vi "gyro-pll-V3.vi"() -> ()   [LabVIEW 2018]
uses:
  lorentzian.ctl
  circle corners.ctl
  pid -- parameters.ctl
  <vilib>/event_ctls.llb/eventvkey.ctl
  show-win- control.ctl
  PID - mode.ctl
  pll parameters.ctl
  server talk-to-back pair.ctl
  server talkback message type.ctl
  server talkto message type.ctl
  agregator -- action.ctl
  interpolation state - real.ctl
  pll internal user event action.ctl
  publisher action.ctl
  four-corner circle transformation.ctl
  cursor action.ctl
  Q -- check range -- i -- real.vi
  linear interpolation - real.vi
  draw a circle.vi
  linear interpolation iiii- complex.vi
  <vilib>/Analysis/baseanly.llb/A x B.vi
  <vilib>/Analysis/baseanly.llb/Complex A x B.vi
  line -- complex.vi
  Q -- check range -- i -- integer.vi
  generate linear region.vi
  Q - not nan -- real.vi
  Q - not nan -- integer.vi
  <vilib>/Analysis/Matrix/Numeric/Conversions/Array To Matrix.vi
  <vilib>/Analysis/Matrix/Numeric/Conversions/Array To Matrix - RA2.vi
  <vilib>/Analysis/baseanly.llb/Inverse Matrix.vi
  <vilib>/Analysis/baseanly.llb/Real Inverse Matrix.vi
panel:
  in  "(*) sweeper server":bool=TRUE
  in  "(*) pll":bool
  in  "exit!":bool
  in  "(*) sourcer":bool
  in  "(*) fitter":bool
  in  "(*) sweeper":bool=TRUE
  in  "PID parameters :{}[];'":T1={"I (sec)"=0.004634123928756344, "P (sec)"=0.008980860327047186} {"P (sec)" scale=0.01..10.0; "I (sec)" scale=0.01..10.0}
  in  "PLL ON":bool
  in  "stop pll async":bool
  in  "start pll async":bool
  in  "pll parameters":T2={"PID parameters"={"I (sec)"=0.004634123928756344, "P (sec)"=0.008980860327047186}, "PID mode"=enum."normal", "plot hist time (sec)"=1.0, "dt (sec)"=0.001, "visc hist time (sec)"=2.0, "time int ave time (sec)"=0.3, "PLL limits (Hz)"=5000.0} {"PLL limits (Hz)" format="%#.2f"; "time int ave time (sec)" format="%#_10f"; "visc hist time (sec)" format="%#_10f"; "dt (sec)" format="%#_10f"; "plot hist time (sec)" format="%#_10f"; "PID parameters"."P (sec)" scale=0.01..10.0; "PID parameters"."I (sec)" scale=0.01..10.0}
  in  "all 3":T4(tab)
  in  "reset lorentzian! :q":bool
  in  "Tab Control":enum32{"PID", "hist", "params"}(tab)=enum."params"
  out "Plot: complex- hist":cluster{dbl[], dbl[]}[](graph)=[{array[1000 elements], array[1000 elements]}, {[7.190597353205284e-06, 7.172141018125027e-06, 7.116804391567491e-06, 7.024684552779172e-06, 6.895943111259833e-06, 6.7308059232445354e-06, 6.529562695475053e-06, 6.292566476955803e-06, 6.020233039585921e-06, 5.713040148754082e-06, 5.371526725175644e-06, 4.996291899442611e-06, 4.5879939609449636e-06, 4.147349203007406e-06, 3.6751306662674513e-06, 3.1721667824994774e-06, 2.6393399212638878e-06, 2.0775848419310813e-06, 1.4878870537958579e-06, 8.712810871592677e-07, 2.2884867841089993e-07, -4.382831277042918e-07, -1.1289439553054788e-06, -1.8419221506129192e-06, -2.575966907600425e-06, -3.329790462334158e-06, -4.102070352148148e-06, -4.891451735693187e-06, -5.696549769788949e-06, -6.515952038909475e-06, -7.348221033039968e-06, -8.191896669557811e-06, -9.045498854713654e-06, -9.907530080218758e-06, -1.0776478050383408e-05, -1.1650818335197432e-05, -1.252901704469844e-05, -1.3409533519936043e-05, -1.4290823035811157e-05, -1.5171339511048758e-05, -1.6049538220549768e-05, -1.692387850536379e-05, -1.7792826475528438e-05, -1.8654857701033543e-05, -1.950845988618939e-05, -2.035213552270723e-05, -2.1184404516837726e-05, -2.200380678595825e-05, -2.2808904820054008e-05, -2.3598286203599055e-05, -2.4370566093413044e-05, -2.5124389648146775e-05, -2.5858434405134282e-05, -2.6571412600441725e-05, -2.7262073428042906e-05, -2.79292052341581e-05, -2.8571637642906468e-05, -2.918824360954306e-05, -2.9777941397678286e-05, -3.0339696477011096e-05, -3.087252333824668e-05, -3.137548722201465e-05, -3.184770575875461e-05, -3.228835051669217e-05, -3.269664845518981e-05, -3.3071883280922845e-05, -3.341339670450129e-05, -3.372058959533313e-05, -3.399292303270301e-05, -3.4229919251222255e-05, -3.4431162478991744e-05, -3.4596299667007035e-05, -3.472504110852638e-05, -3.4817160947314696e-05, -3.4872497573872235e-05, -3.489095390895249e-05, -3.4872497573872235e-05, -3.4817160947314696e-05, -3.472504110852638e-05, -3.459629966700704e-05, -3.4431162478991744e-05, -3.422991925122226e-05, -3.3992923032703014e-05, -3.372058959533313e-05, -3.341339670450129e-05, -3.307188328092285e-05, -3.269664845518982e-05, -3.2288350516692175e-05, -3.1847705758754615e-05, -3.137548722201466e-05, -3.087252333824669e-05, -3.0339696477011103e-05, -2.9777941397678293e-05, -2.9188243609543066e-05, -2.8571637642906474e-05, -2.7929205234158112e-05, -2.726207342804292e-05, -2.6571412600441735e-05, -2.5858434405134296e-05, -2.512438964814679e-05, -2.4370566093413057e-05, -2.3598286203599066e-05, -2.280890482005402e-05, -2.200380678595826e-05, -2.1184404516837737e-05, -2.035213552270724e-05, -1.9508459886189396e-05, -1.865485770103357e-05, -1.7792826475528462e-05, -1.6923878505363813e-05, -1.6049538220549788e-05, -1.5171339511048779e-05, -1.4290823035811176e-05, -1.3409533519936056e-05, -1.2529017044698455e-05, -1.1650818335197446e-05, -1.0776478050383421e-05, -9.907530080218769e-06, -9.045498854713664e-06, -8.19189666955782e-06, -7.348221033039972e-06, -6.515952038909498e-06, -5.69654976978897e-06, -4.891451735693207e-06, -4.102070352148165e-06, -3.3297904623341733e-06, -2.575966907600442e-06, -1.8419221506129327e-06, -1.1289439553054907e-06, -4.3828312770430365e-07, 2.2884867841089146e-07, 8.712810871592576e-07, 1.4878870537958511e-06, 2.0775848419310745e-06, 2.6393399212638844e-06, 3.172166782499474e-06, 3.6751306662674378e-06, 4.147349203007396e-06, 4.587993960944957e-06, 4.996291899442601e-06, 5.371526725175637e-06, 5.713040148754075e-06, 6.020233039585914e-06, 6.292566476955799e-06, 6.52956269547505e-06, 6.7308059232445354e-06, 6.89594311125983e-06, 7.024684552779168e-06, 7.116804391567491e-06, 7.172141018125027e-06], [0.0002113633008955132, 0.00021224439713003404, 0.00021312394762236102, 0.00021400040934205735, 0.00021487224467744295, 0.00021573792413308792, 0.00021659592901306725, 0.0002174447540852694, 0.00021828291022208502, 0.0002191089270128428, 0.00021992135534340933, 0.00022071876993842783, 0.00022149977186173528, 0.00022226299097057205, 0.00022300708831927754, 0.00022373075850825623, 0.00022443273197409182, 0.00022511177721679307, 0.00022576670296026313, 0.00022639636024220273, 0.00022699964442978034, 0.0002275754971575336, 0.000228122908184102, 0.00022864091716453335, 0.0002291286153350554, 0.0002295851471073561, 0.00023000971156957625, 0.00023040156389138116, 0.0002307600166306461, 0.00023108444093946333, 0.00023137426766735506, 0.00023162898835975677, 0.0002318481561500193, 0.00023203138654336486, 0.0002321783580914214, 0.00023228881295615236, 0.00023236255736219216, 0.00023239946193679412, 0.00023239946193679412, 0.00023236255736219216, 0.00023228881295615236, 0.0002321783580914214, 0.00023203138654336486, 0.0002318481561500193, 0.00023162898835975677, 0.00023137426766735506, 0.00023108444093946333, 0.00023076001663064613, 0.00023040156389138116, 0.00023000971156957625, 0.0002295851471073561, 0.0002291286153350554, 0.00022864091716453335, 0.000228122908184102, 0.0002275754971575336, 0.00022699964442978034, 0.00022639636024220273, 0.00022576670296026315, 0.00022511177721679307, 0.00022443273197409182, 0.00022373075850825623, 0.00022300708831927757, 0.00022226299097057205, 0.0002214997718617353, 0.00022071876993842783, 0.00021992135534340933, 0.0002191089270128428, 0.00021828291022208502, 0.0002174447540852694, 0.00021659592901306725, 0.00021573792413308792, 0.00021487224467744295, 0.00021400040934205735, 0.00021312394762236102, 0.00021224439713003404, 0.0002113633008955132, 0.00021048220466099237, 0.0002096026541686654, 0.0002087261924489691, 0.0002078543571135835, 0.0002069886776579385, 0.00020613067277795916, 0.00020528184770575705, 0.00020444369156894142, 0.00020361767477818362, 0.00020280524644761708, 0.0002020078318525986, 0.00020122682992929113, 0.0002004636108204544, 0.00019971951347174887, 0.00019899584328277018, 0.0001982938698169346, 0.00019761482457423337, 0.0001969598988307633, 0.00019633024154882368, 0.00019572695736124607, 0.0001951511046334928, 0.00019460369360692445, 0.00019408568462649307, 0.00019359798645597102, 0.00019314145468367035, 0.0001927168902214502, 0.00019232503789964525, 0.0001919665851603803, 0.00019164216085156309, 0.00019135233412367135, 0.00019109761343126964, 0.0001908784456410071, 0.00019069521524766155, 0.000190548243699605, 0.00019043778883487406, 0.00019036404442883425, 0.0001903271398542323, 0.0001903271398542323, 0.00019036404442883425, 0.00019043778883487406, 0.000190548243699605, 0.00019069521524766155, 0.0001908784456410071, 0.00019109761343126964, 0.00019135233412367135, 0.00019164216085156306, 0.00019196658516038029, 0.00019232503789964523, 0.00019271689022145016, 0.00019314145468367033, 0.000193597986455971, 0.00019408568462649307, 0.00019460369360692443, 0.0001951511046334928, 0.00019572695736124607, 0.00019633024154882368, 0.00019695989883076326, 0.00019761482457423334, 0.0001982938698169346, 0.00019899584328277018, 0.00019971951347174885, 0.00020046361082045436, 0.0002012268299292911, 0.00020200783185259858, 0.00020280524644761705, 0.0002036176747781836, 0.0002044436915689414, 0.00020528184770575702, 0.00020613067277795916, 0.0002069886776579385, 0.00020785435711358346, 0.00020872619244896907, 0.00020960265416866537, 0.00021048220466099237]}, {[7.168586400274939e-06, 5.066709932460086e-06, 2.964833464645231e-06, 8.629569968303764e-07, -1.2389194709844774e-06, -3.340795938799331e-06, -5.442672406614187e-06, -7.54454887442904e-06, -9.646425342243894e-06, -1.174830181005875e-05, -1.3850178277873602e-05, -1.5952054745688457e-05, -1.8053931213503313e-05, -2.0155807681318165e-05, -2.225768414913302e-05, -2.4359560616947872e-05, -2.6461437084762728e-05, -2.8563313552577583e-05, -3.066519002039244e-05, -3.276706648820729e-05], [0.00021232547061132137, 0.00021222925363974056, 0.00021213303666815973, 0.00021203681969657892, 0.0002119406027249981, 0.0002118443857534173, 0.00021174816878183648, 0.00021165195181025565, 0.00021155573483867484, 0.000211459517867094, 0.0002113633008955132, 0.0002112670839239324, 0.00021117086695235157, 0.00021107464998077076, 0.00021097843300918993, 0.00021088221603760913, 0.00021078599906602832, 0.0002106897820944475, 0.00021059356512286668, 0.00021049734815128585]}, {[-1.288800856206544e-05, -1.2984225533646258e-05, -1.3080442505227073e-05, -1.317665947680789e-05, -1.3272876448388706e-05, -1.3369093419969523e-05, -1.3465310391550338e-05, -1.3561527363131155e-05, -1.365774433471197e-05, -1.3753961306292788e-05, -1.3850178277873605e-05, -1.394639524945442e-05, -1.4042612221035236e-05, -1.4138829192616053e-05, -1.423504616419687e-05, -1.4331263135777686e-05, -1.4427480107358503e-05, -1.4523697078939318e-05, -1.4619914050520135e-05, -1.471613102210095e-05], [0.00019034453621736468, 0.00019244641268517952, 0.0001945482891529944, 0.00019665016562080923, 0.0001987520420886241, 0.00020085391855643894, 0.00020295579502425378, 0.00020505767149206865, 0.0002071595479598835, 0.00020926142442769836, 0.0002113633008955132, 0.00021346517736332805, 0.00021556705383114292, 0.00021766893029895776, 0.00021977080676677263, 0.00022187268323458747, 0.0002239745597024023, 0.00022607643617021718, 0.00022817831263803202, 0.0002302801891058469]}, {[9.092925831891258e-06, 8.900491888729626e-06, 8.708057945567993e-06, 8.515624002406362e-06, 8.32319005924473e-06, 8.130756116083097e-06, 7.938322172921465e-06, 7.745888229759832e-06, 7.5534542865982e-06, 7.361020343436568e-06, 7.168586400274936e-06, 6.976152457113303e-06, 6.783718513951671e-06, 6.591284570790038e-06, 6.3988506276284065e-06, 6.206416684466774e-06, 6.013982741305142e-06, 5.82154879814351e-06, 5.629114854981877e-06, 5.4366809118202445e-06], [0.0001702879412550243, 0.00017449169419065402, 0.00017869544712628373, 0.00018289920006191342, 0.00018710295299754313, 0.00019130670593317284, 0.00019551045886880255, 0.00019971421180443226, 0.00020391796474006197, 0.00020812171767569168, 0.00021232547061132137, 0.00021652922354695108, 0.0002207329764825808, 0.0002249367294182105, 0.0002291404823538402, 0.0002333442352894699, 0.00023754798822509963, 0.00024175174116072932, 0.00024595549409635905, 0.00025015924703198874]}, {[-1.97103396318906e-05, -1.91243234964889e-05, -1.8538307361087202e-05, -1.79522912256855e-05, -1.73662750902838e-05, -1.6780258954882103e-05, -1.6194242819480402e-05, -1.5608226684078704e-05, -1.5022210548677003e-05, -1.4436194413275303e-05, -1.3850178277873603e-05, -1.3264162142471904e-05, -1.2678146007070203e-05, -1.2092129871668504e-05, -1.1506113736266805e-05, -1.0920097600865104e-05, -1.0334081465463405e-05, -9.748065330061706e-06, -9.162049194660005e-06, -8.576033059258306e-06], [0.00023375398508080204, 0.00023151491666227315, 0.00022927584824374426, 0.0002270367798252154, 0.0002247977114066865, 0.00022255864298815762, 0.00022031957456962873, 0.00021808050615109985, 0.00021584143773257098, 0.0002136023693140421, 0.0002113633008955132, 0.00020912423247698432, 0.00020688516405845543, 0.00020464609563992657, 0.00020240702722139768, 0.0002001679588028688, 0.0001979288903843399, 0.00019568982196581104, 0.00019345075354728215, 0.00019121168512875326]}]
  in  "dt (sec)":dbl=0.001 format="%#_10f"
  in  "plot hist time (sec)":dbl=1.0 format="%#_10f"
  in  "PID mode":T3
  out "G (Hz)":dbl=6.817921124952451 format="%#.4f"
  in  "reset freq! :r":bool
  out "Plot: complex plane":cluster{dbl[], dbl[]}[](graph)=[{[7.190597353205284e-06, 7.172141018125027e-06, 7.116804391567491e-06, 7.024684552779172e-06, 6.895943111259833e-06, 6.7308059232445354e-06, 6.529562695475053e-06, 6.292566476955803e-06, 6.020233039585921e-06, 5.713040148754082e-06, 5.371526725175644e-06, 4.996291899442611e-06, 4.5879939609449636e-06, 4.147349203007406e-06, 3.6751306662674513e-06, 3.1721667824994774e-06, 2.6393399212638878e-06, 2.0775848419310813e-06, 1.4878870537958579e-06, 8.712810871592677e-07, 2.2884867841089993e-07, -4.382831277042918e-07, -1.1289439553054788e-06, -1.8419221506129192e-06, -2.575966907600425e-06, -3.329790462334158e-06, -4.102070352148148e-06, -4.891451735693187e-06, -5.696549769788949e-06, -6.515952038909475e-06, -7.348221033039968e-06, -8.191896669557811e-06, -9.045498854713654e-06, -9.907530080218758e-06, -1.0776478050383408e-05, -1.1650818335197432e-05, -1.252901704469844e-05, -1.3409533519936043e-05, -1.4290823035811157e-05, -1.5171339511048758e-05, -1.6049538220549768e-05, -1.692387850536379e-05, -1.7792826475528438e-05, -1.8654857701033543e-05, -1.950845988618939e-05, -2.035213552270723e-05, -2.1184404516837726e-05, -2.200380678595825e-05, -2.2808904820054008e-05, -2.3598286203599055e-05, -2.4370566093413044e-05, -2.5124389648146775e-05, -2.5858434405134282e-05, -2.6571412600441725e-05, -2.7262073428042906e-05, -2.79292052341581e-05, -2.8571637642906468e-05, -2.918824360954306e-05, -2.9777941397678286e-05, -3.0339696477011096e-05, -3.087252333824668e-05, -3.137548722201465e-05, -3.184770575875461e-05, -3.228835051669217e-05, -3.269664845518981e-05, -3.3071883280922845e-05, -3.341339670450129e-05, -3.372058959533313e-05, -3.399292303270301e-05, -3.4229919251222255e-05, -3.4431162478991744e-05, -3.4596299667007035e-05, -3.472504110852638e-05, -3.4817160947314696e-05, -3.4872497573872235e-05, -3.489095390895249e-05, -3.4872497573872235e-05, -3.4817160947314696e-05, -3.472504110852638e-05, -3.459629966700704e-05, -3.4431162478991744e-05, -3.422991925122226e-05, -3.3992923032703014e-05, -3.372058959533313e-05, -3.341339670450129e-05, -3.307188328092285e-05, -3.269664845518982e-05, -3.2288350516692175e-05, -3.1847705758754615e-05, -3.137548722201466e-05, -3.087252333824669e-05, -3.0339696477011103e-05, -2.9777941397678293e-05, -2.9188243609543066e-05, -2.8571637642906474e-05, -2.7929205234158112e-05, -2.726207342804292e-05, -2.6571412600441735e-05, -2.5858434405134296e-05, -2.512438964814679e-05, -2.4370566093413057e-05, -2.3598286203599066e-05, -2.280890482005402e-05, -2.200380678595826e-05, -2.1184404516837737e-05, -2.035213552270724e-05, -1.9508459886189396e-05, -1.865485770103357e-05, -1.7792826475528462e-05, -1.6923878505363813e-05, -1.6049538220549788e-05, -1.5171339511048779e-05, -1.4290823035811176e-05, -1.3409533519936056e-05, -1.2529017044698455e-05, -1.1650818335197446e-05, -1.0776478050383421e-05, -9.907530080218769e-06, -9.045498854713664e-06, -8.19189666955782e-06, -7.348221033039972e-06, -6.515952038909498e-06, -5.69654976978897e-06, -4.891451735693207e-06, -4.102070352148165e-06, -3.3297904623341733e-06, -2.575966907600442e-06, -1.8419221506129327e-06, -1.1289439553054907e-06, -4.3828312770430365e-07, 2.2884867841089146e-07, 8.712810871592576e-07, 1.4878870537958511e-06, 2.0775848419310745e-06, 2.6393399212638844e-06, 3.172166782499474e-06, 3.6751306662674378e-06, 4.147349203007396e-06, 4.587993960944957e-06, 4.996291899442601e-06, 5.371526725175637e-06, 5.713040148754075e-06, 6.020233039585914e-06, 6.292566476955799e-06, 6.52956269547505e-06, 6.7308059232445354e-06, 6.89594311125983e-06, 7.024684552779168e-06, 7.116804391567491e-06, 7.172141018125027e-06], [0.0002113633008955132, 0.00021224439713003404, 0.00021312394762236102, 0.00021400040934205735, 0.00021487224467744295, 0.00021573792413308792, 0.00021659592901306725, 0.0002174447540852694, 0.00021828291022208502, 0.0002191089270128428, 0.00021992135534340933, 0.00022071876993842783, 0.00022149977186173528, 0.00022226299097057205, 0.00022300708831927754, 0.00022373075850825623, 0.00022443273197409182, 0.00022511177721679307, 0.00022576670296026313, 0.00022639636024220273, 0.00022699964442978034, 0.0002275754971575336, 0.000228122908184102, 0.00022864091716453335, 0.0002291286153350554, 0.0002295851471073561, 0.00023000971156957625, 0.00023040156389138116, 0.0002307600166306461, 0.00023108444093946333, 0.00023137426766735506, 0.00023162898835975677, 0.0002318481561500193, 0.00023203138654336486, 0.0002321783580914214, 0.00023228881295615236, 0.00023236255736219216, 0.00023239946193679412, 0.00023239946193679412, 0.00023236255736219216, 0.00023228881295615236, 0.0002321783580914214, 0.00023203138654336486, 0.0002318481561500193, 0.00023162898835975677, 0.00023137426766735506, 0.00023108444093946333, 0.00023076001663064613, 0.00023040156389138116, 0.00023000971156957625, 0.0002295851471073561, 0.0002291286153350554, 0.00022864091716453335, 0.000228122908184102, 0.0002275754971575336, 0.00022699964442978034, 0.00022639636024220273, 0.00022576670296026315, 0.00022511177721679307, 0.00022443273197409182, 0.00022373075850825623, 0.00022300708831927757, 0.00022226299097057205, 0.0002214997718617353, 0.00022071876993842783, 0.00021992135534340933, 0.0002191089270128428, 0.00021828291022208502, 0.0002174447540852694, 0.00021659592901306725, 0.00021573792413308792, 0.00021487224467744295, 0.00021400040934205735, 0.00021312394762236102, 0.00021224439713003404, 0.0002113633008955132, 0.00021048220466099237, 0.0002096026541686654, 0.0002087261924489691, 0.0002078543571135835, 0.0002069886776579385, 0.00020613067277795916, 0.00020528184770575705, 0.00020444369156894142, 0.00020361767477818362, 0.00020280524644761708, 0.0002020078318525986, 0.00020122682992929113, 0.0002004636108204544, 0.00019971951347174887, 0.00019899584328277018, 0.0001982938698169346, 0.00019761482457423337, 0.0001969598988307633, 0.00019633024154882368, 0.00019572695736124607, 0.0001951511046334928, 0.00019460369360692445, 0.00019408568462649307, 0.00019359798645597102, 0.00019314145468367035, 0.0001927168902214502, 0.00019232503789964525, 0.0001919665851603803, 0.00019164216085156309, 0.00019135233412367135, 0.00019109761343126964, 0.0001908784456410071, 0.00019069521524766155, 0.000190548243699605, 0.00019043778883487406, 0.00019036404442883425, 0.0001903271398542323, 0.0001903271398542323, 0.00019036404442883425, 0.00019043778883487406, 0.000190548243699605, 0.00019069521524766155, 0.0001908784456410071, 0.00019109761343126964, 0.00019135233412367135, 0.00019164216085156306, 0.00019196658516038029, 0.00019232503789964523, 0.00019271689022145016, 0.00019314145468367033, 0.000193597986455971, 0.00019408568462649307, 0.00019460369360692443, 0.0001951511046334928, 0.00019572695736124607, 0.00019633024154882368, 0.00019695989883076326, 0.00019761482457423334, 0.0001982938698169346, 0.00019899584328277018, 0.00019971951347174885, 0.00020046361082045436, 0.0002012268299292911, 0.00020200783185259858, 0.00020280524644761705, 0.0002036176747781836, 0.0002044436915689414, 0.00020528184770575702, 0.00020613067277795916, 0.0002069886776579385, 0.00020785435711358346, 0.00020872619244896907, 0.00020960265416866537, 0.00021048220466099237]}, {[7.168586400274939e-06, 5.066709932460086e-06, 2.964833464645231e-06, 8.629569968303764e-07, -1.2389194709844774e-06, -3.340795938799331e-06, -5.442672406614187e-06, -7.54454887442904e-06, -9.646425342243894e-06, -1.174830181005875e-05, -1.3850178277873602e-05, -1.5952054745688457e-05, -1.8053931213503313e-05, -2.0155807681318165e-05, -2.225768414913302e-05, -2.4359560616947872e-05, -2.6461437084762728e-05, -2.8563313552577583e-05, -3.066519002039244e-05, -3.276706648820729e-05], [0.00021232547061132137, 0.00021222925363974056, 0.00021213303666815973, 0.00021203681969657892, 0.0002119406027249981, 0.0002118443857534173, 0.00021174816878183648, 0.00021165195181025565, 0.00021155573483867484, 0.000211459517867094, 0.0002113633008955132, 0.0002112670839239324, 0.00021117086695235157, 0.00021107464998077076, 0.00021097843300918993, 0.00021088221603760913, 0.00021078599906602832, 0.0002106897820944475, 0.00021059356512286668, 0.00021049734815128585]}, {[-1.288800856206544e-05, -1.2984225533646258e-05, -1.3080442505227073e-05, -1.317665947680789e-05, -1.3272876448388706e-05, -1.3369093419969523e-05, -1.3465310391550338e-05, -1.3561527363131155e-05, -1.365774433471197e-05, -1.3753961306292788e-05, -1.3850178277873605e-05, -1.394639524945442e-05, -1.4042612221035236e-05, -1.4138829192616053e-05, -1.423504616419687e-05, -1.4331263135777686e-05, -1.4427480107358503e-05, -1.4523697078939318e-05, -1.4619914050520135e-05, -1.471613102210095e-05], [0.00019034453621736468, 0.00019244641268517952, 0.0001945482891529944, 0.00019665016562080923, 0.0001987520420886241, 0.00020085391855643894, 0.00020295579502425378, 0.00020505767149206865, 0.0002071595479598835, 0.00020926142442769836, 0.0002113633008955132, 0.00021346517736332805, 0.00021556705383114292, 0.00021766893029895776, 0.00021977080676677263, 0.00022187268323458747, 0.0002239745597024023, 0.00022607643617021718, 0.00022817831263803202, 0.0002302801891058469]}, {[9.092925831891258e-06, 8.900491888729626e-06, 8.708057945567993e-06, 8.515624002406362e-06, 8.32319005924473e-06, 8.130756116083097e-06, 7.938322172921465e-06, 7.745888229759832e-06, 7.5534542865982e-06, 7.361020343436568e-06, 7.168586400274936e-06, 6.976152457113303e-06, 6.783718513951671e-06, 6.591284570790038e-06, 6.3988506276284065e-06, 6.206416684466774e-06, 6.013982741305142e-06, 5.82154879814351e-06, 5.629114854981877e-06, 5.4366809118202445e-06], [0.0001702879412550243, 0.00017449169419065402, 0.00017869544712628373, 0.00018289920006191342, 0.00018710295299754313, 0.00019130670593317284, 0.00019551045886880255, 0.00019971421180443226, 0.00020391796474006197, 0.00020812171767569168, 0.00021232547061132137, 0.00021652922354695108, 0.0002207329764825808, 0.0002249367294182105, 0.0002291404823538402, 0.0002333442352894699, 0.00023754798822509963, 0.00024175174116072932, 0.00024595549409635905, 0.00025015924703198874]}]
  in  "lorentzian":T5={"A (VHz)"=0.0007250653088846297, "f (Hz)"=45017.43809779818, "G (Hz)"=34.46000858512321, "phi(rad)"=-1.525051560312372, "Q"=1306.3675821959234, "Norm  Ampl"=nan, "bg (V)"=7.168586400274938e-06+0.00021232547061132137i, "4corners"={"z (-pi/2)"=-1.288800856206544e-05+0.00019034453621736468i, "z(inf)"=7.168586400274938e-06+0.00021232547061132137i, "z (pi/2)"=-1.4812347993681768e-05+0.00023238206557366173i, "z center"=-1.3850178277873603e-05+0.0002113633008955132i, "z(0)"=-3.486894295602214e-05+0.00021040113117970505i, "radius"=2.1040775631078887e-05}} {"bg (V)" format="%#9_9f"; "Q" format="%#9_9f"; "phi(rad)" format="%#9_9f"; "G (Hz)" format="%#9_9f"; "f (Hz)" format="%#9_9f"}
  in  "toggle PLL! :@":bool
  out "f (Hz)":dbl=40017.438097734725 format="%#.11f"
  out "VKey":T7
  out "Char":i16=62
  in  "lorentzian -- basic":T5={"A (VHz)"=1.0, "f (Hz)"=1000.0, "G (Hz)"=3.0, "phi(rad)"=0.0, "Q"=300.0, "Norm  Ampl"=nan, "bg (V)"=0.0+0.0i, "4corners"={"z (-pi/2)"=9.277908004825974e-07+0.0007240755403629966i, "z(inf)"=2.6527949823343002e-05+0.0007477540585896028i, "z (pi/2)"=2.8494315967368497e-06+0.0007733542176124632i, "z center"=1.8886111986097237e-06+0.0007487148789877299i, "z(0)"=-2.2750727426123552e-05+0.000749675699385857i, "radius"=2.4658065287076567e-05}} {"bg (V)" format="%#9_9f"; "Q" format="%#9_9f"; "phi(rad)" format="%#9_9f"; "G (Hz)" format="%#9_9f"; "f (Hz)" format="%#9_9f"}
  in  "save lor for later":bool
  in  "reset lorentzian from basic":bool
  out "zi out Im (V)":dbl=-2.55535250615244e-07 format="%#.8f"
  out "zi out Re (V)":dbl=2.3785838016890924e-07 format="%#.8f"
  out "publish message":T8
  out "window":T9={"cen (Hz)"=45496.74569300777, "win (Hz)"=29.962105514646385, "left (Hz)"=45481.76464025045, "right (Hz)"=45511.72674576509}
  in  "lorentzian -- hist":T5={"A (VHz)"=0.0007250653088846297, "f (Hz)"=45017.43809779818, "G (Hz)"=34.46000858512321, "phi(rad)"=-1.525051560312372, "Q"=1306.3675821959234, "Norm  Ampl"=nan, "bg (V)"=7.168586400274938e-06+0.00021232547061132137i, "4corners"={"z (-pi/2)"=-1.288800856206544e-05+0.00019034453621736468i, "z(inf)"=7.168586400274938e-06+0.00021232547061132137i, "z (pi/2)"=-1.4812347993681768e-05+0.00023238206557366173i, "z center"=-1.3850178277873603e-05+0.0002113633008955132i, "z(0)"=-3.486894295602214e-05+0.00021040113117970505i, "radius"=2.1040775631078887e-05}} {"bg (V)" format="%#9_9f"; "Q" format="%#9_9f"; "phi(rad)" format="%#9_9f"; "G (Hz)" format="%#9_9f"; "f (Hz)" format="%#9_9f"}
  out "pll event pair":T10
  out "sweeper server reference":refnum<vi>
  out "pll async reference":refnum<vi>
  out "async fitter":refnum<vi>
  out "async sweeper":refnum<vi>
  out "fitter event pair":T10
  out "sweeper event pair":T10
  out "async sourcer":refnum<vi>
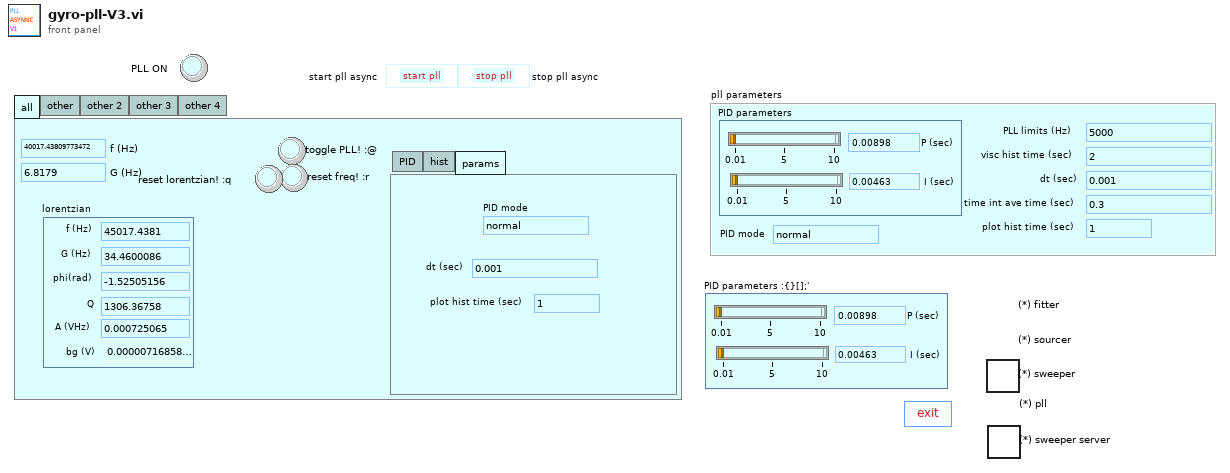
[diagram p1: front panel]
types:
  T1 = typedef "pid -- parameters.ctl" = cluster{"I (sec)":dbl, "P (sec)":dbl}
  T2 = typedef "pll parameters.ctl" = cluster{"PID parameters":T1, "PID mode":T3, "plot hist time (sec)":dbl, "dt (sec)":dbl, "visc hist time (sec)":dbl, "time int ave time (sec)":dbl, "PLL limits (Hz)":dbl}
  T3 = typedef "PID - mode.ctl" = enum16{"normal", "heat"}
  T4 = enum32{"all", "other", "other 2", "other 3", "other 4"}
  T5 = typedef "lorentzian.ctl" = cluster{"A (VHz)":dbl, "f (Hz)":dbl, "G (Hz)":dbl, "phi(rad)":dbl, "Q":dbl, "Norm  Ampl":dbl, "bg (V)":cdb, "4corners":T6}
  T6 = typedef "circle corners.ctl" = cluster{"z (-pi/2)":cdb, "z(inf)":cdb, "z (pi/2)":cdb, "z center":cdb, "z(0)":cdb, "radius":dbl}
  T7 = typedef "eventvkey.ctl" = enum16{"ASCII", "Enter", "Return", "Shift", "Ctrl", "Alt", "Cmd", "Opt", "Caps", "NumLock", "Clear", "Break", "Up", "Down", "Left", "Right", "Insert", "Delete", "Home", "End", "PageUp", "PageDown", "Escape", "Help", "Pause", "ScrollLock", "F1", "F2", "F3", "F4", "F5", "F6", "F7", "F8", "F9", "F10", "F11", "F12", "F13", "F14", "F15", "F16", "F17", "F18", "F19", "F20", "F21", "F22", "F23", "F24", "Play", "VolumeUp", "VolumeDown", "Mute", "Two Byte Char"}
  T8 = cluster{"freq (Hz)":dbl, "gamma (Hz)":dbl, "Voltage (V)":cdb}
  T9 = typedef "show-win- control.ctl" = cluster{"cen (Hz)":dbl, "win (Hz)":dbl, "left (Hz)":dbl, "right (Hz)":dbl}
  T10 = typedef "server talk-to-back pair.ctl" = cluster{"talkback event":refnum<user-event>, "talkto event":refnum<user-event>}
  T11 = typedef "server talkback message type.ctl" = cluster{"message":enum16{"new", "void"}}
  T12 = typedef "server talkto message type.ctl" = cluster{"message":enum16{"stop", "start", "update pars", "update request", "new", "launch", "exit", "get", "reset", "pause", "unpause"}}
  T13 = typedef "pll internal user event action.ctl" = enum16{"gear pll async", "start pll async", "stop pll async", "toggle pll async", "gear sweeper", "start sweeper", "stop sweeper", "toggle sweeper", "accept frequency", "reset lorentzian", "accept lorentzian", "update cursors", "pause pll", "unpause pll", "void", "exit", "gear server sweeper", "gear sweeper async", "gear fitter", "gear sourcer"}
  T14 = typedef "interpolation state - real.ctl" = cluster{"requested size":i32, "Array":dbl[], "actual number of elements":i32}
  T15 = typedef "agregator -- action.ctl" = enum16{"append", "interpolate", "empty!", "force", "init", "scale", "read last"}
  T16 = typedef "publisher action.ctl" = enum16{"set", "get", "init", "check"}
  T17 = typedef "cursor action.ctl" = enum16{"range", "read", "write", "check", "zoom out", "smart zoom out", "zoom to aspect ratio 1", "zoom to win", "zoom out 20%", "zoom in 20%", "-empty", "smart zoom out&aspect", "move range left 20%", "move range right 20%", "move range up 20%", "move range down 20%", "zoom to X win", "zoom to Y win", "zoom out X", "zoom out Y", "zoom in X", "zoom in Y", "check plot scale"}
  T18 = typedef "four-corner circle transformation.ctl" = enum16{"z(c) z(inf)", "z(c) z(zero)", "fix phase", "calculate lorentzian", "z(0) z(+-pi/2)", "shift to zcenter", "to  canonical", "get canonical phase", "get4corners", "update lorentzian -- from z0", "fake gamma normal", "fake gamma heat", "calculate complex slope"}
  T19 = typedef "pll talkback data type.ctl" = cluster{"freq (Hz)":dbl, "gamma (Hz)":dbl, "Voltage (V)":cdb, "overlimit ?":bool}
  T20 = typedef "interpolation state - complex.ctl" = cluster{"requested size":i32, "Array":cdb[], "actual number of elements":i32}
  T21 = enum32{"Invalid", "Standard", "Closed", "Hidden", "Minimized", "Maximized"}
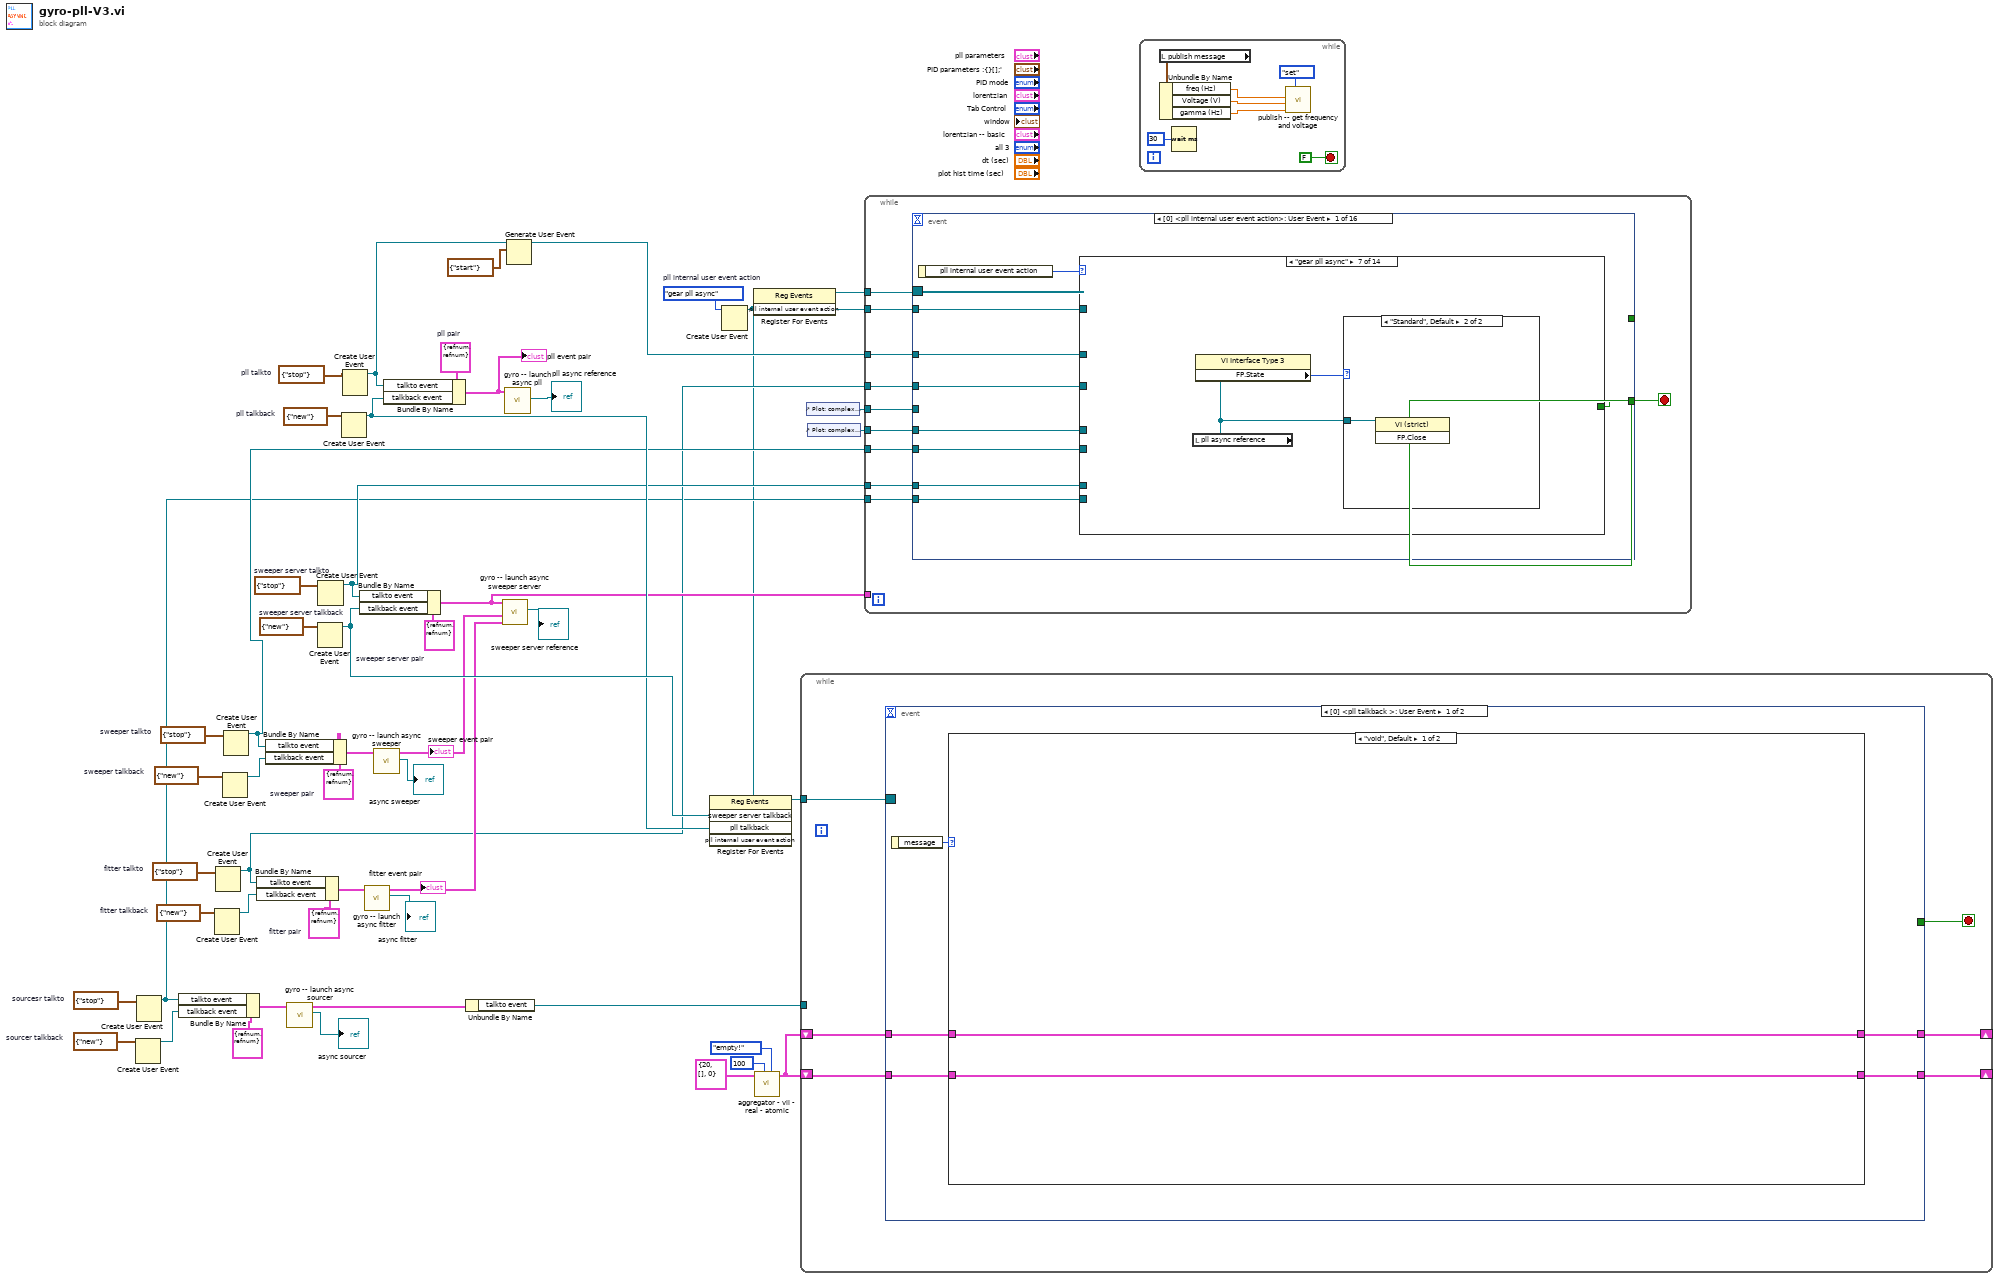
[diagram p0: block diagram]
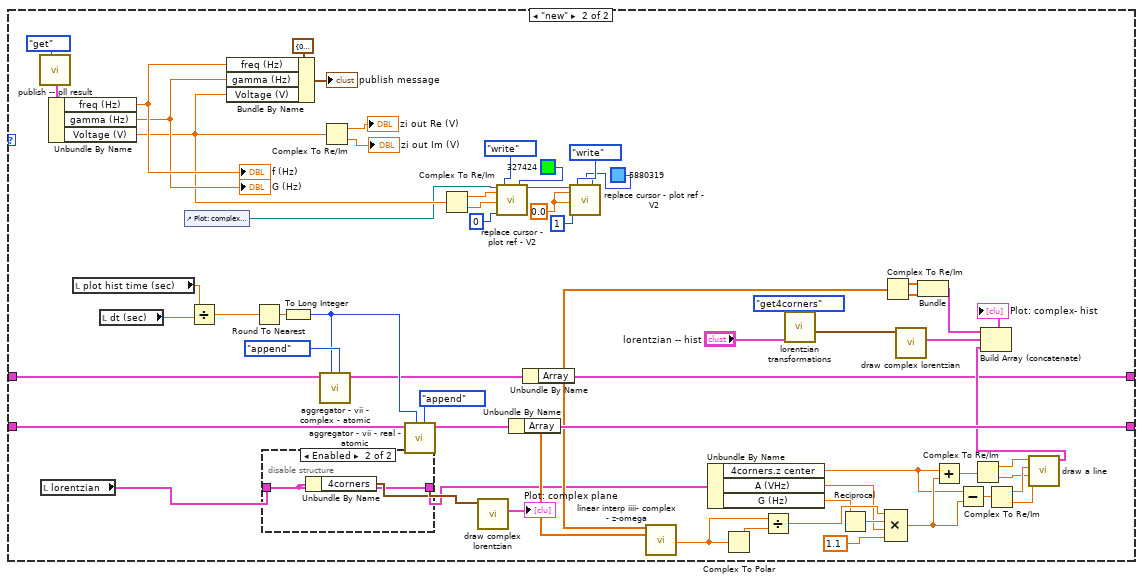
[diagram p2: hidden frame]
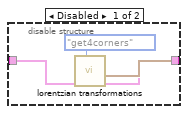
[diagram p3: hidden frame]
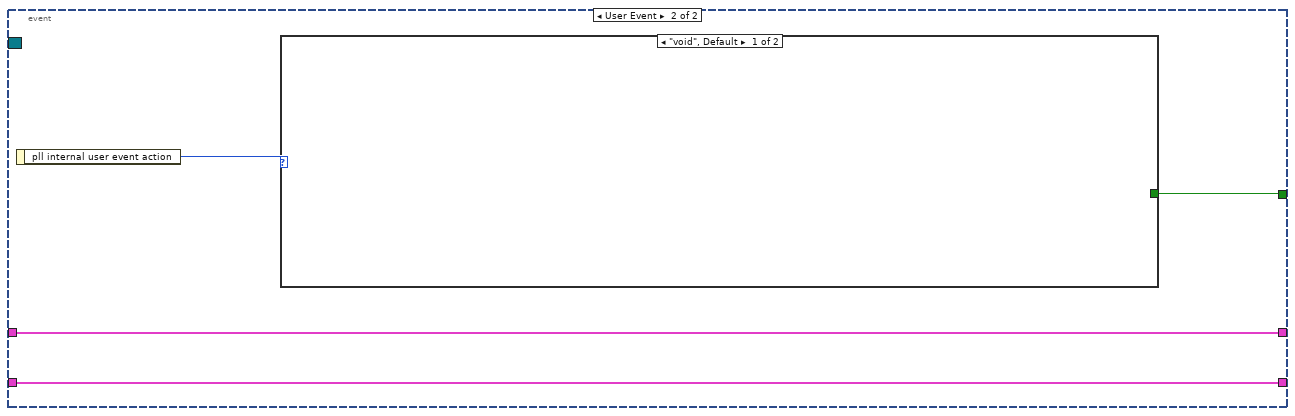
[diagram p4: hidden frame]
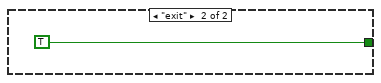
[diagram p5: hidden frame]
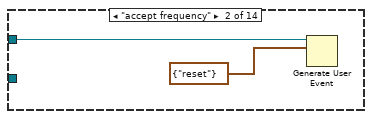
[diagram p7: hidden frame]
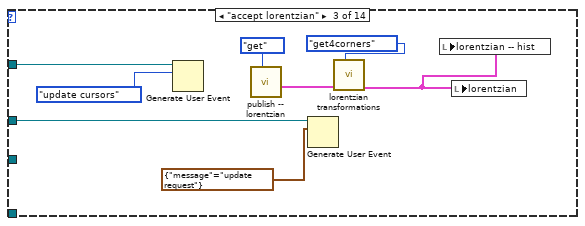
[diagram p8: hidden frame]
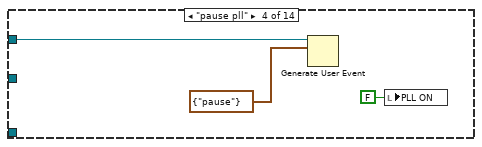
[diagram p9: hidden frame]
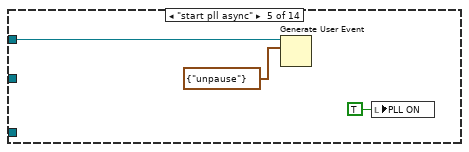
[diagram p10: hidden frame]
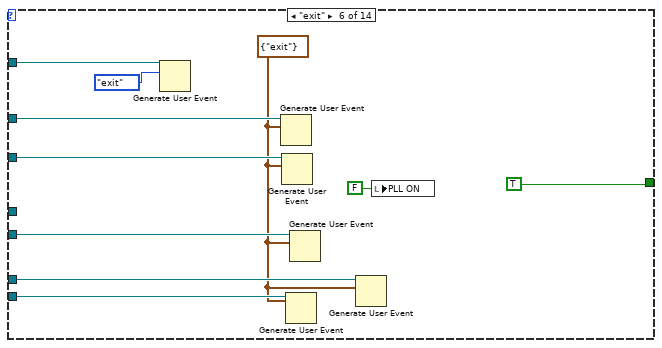
[diagram p11: hidden frame]
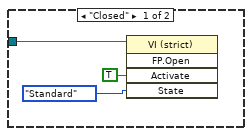
[diagram p12: hidden frame]
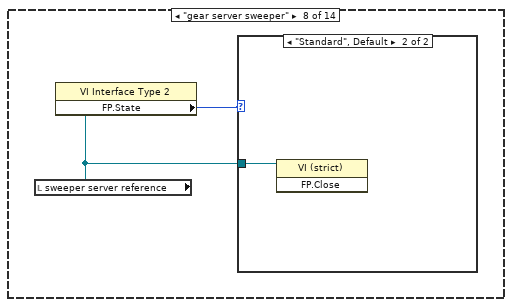
[diagram p13: hidden frame]
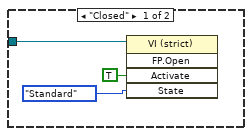
[diagram p14: hidden frame]
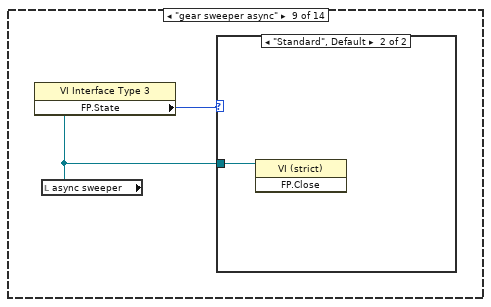
[diagram p15: hidden frame]
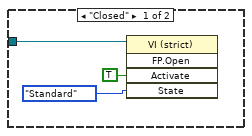
[diagram p16: hidden frame]
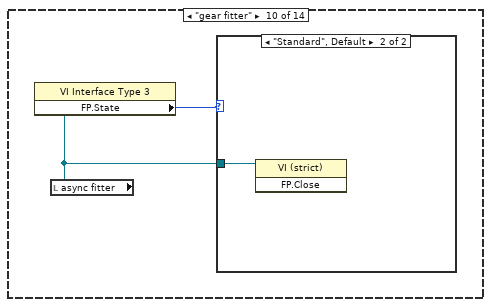
[diagram p17: hidden frame]
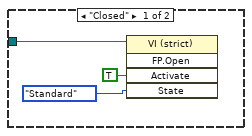
[diagram p18: hidden frame]
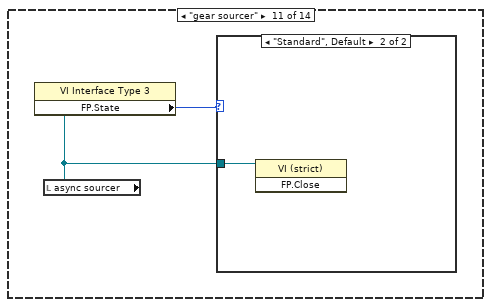
[diagram p19: hidden frame]
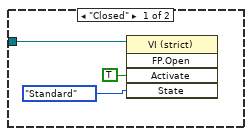
[diagram p20: hidden frame]
diagram:
  w10 = T11 {"message"=enum."new"}  # sourcer talkback
  w11 = T12 {"message"=enum."stop"}  # sourcesr talkto
  w23 = T10 {"talkback event"=refnum, "talkto event"=refnum}  # pll pair
  w21 = T11 {"message"=enum."new"}  # pll talkback
  w22 = T12 {"message"=enum."stop"}  # pll talkto
  w30 = T10 {"talkback event"=refnum, "talkto event"=refnum}  # sweeper server pair
  w28 = T11 {"message"=enum."new"}  # sweeper server talkback
  w29 = T12 {"message"=enum."stop"}  # sweeper server talkto
  w39 = T10 {"talkback event"=refnum, "talkto event"=refnum}  # sweeper pair
  w35 = T11 {"message"=enum."new"}  # sweeper talkback
  w36 = T12 {"message"=enum."stop"}  # sweeper talkto
  w40 = T10 {"talkback event"=refnum, "talkto event"=refnum}  # fitter pair
  w33 = T11 {"message"=enum."new"}  # fitter talkback
  w34 = T12 {"message"=enum."stop"}  # fitter talkto
  w43 = pll_internal_user_event_action."gear pll async"  # pll internal user event action
  n1 = Create User Event(user event datatype=w10) -> (user event=w8:refnum<user-event>)  [unwired: 1 in, 1 out]
  n2 = Create User Event(user event datatype=w11) -> (user event=w2:refnum<user-event>)  [unwired: 1 in, 1 out]
  n3 = Bundle By Name(cluster=T10 {"talkback event"=refnum, "talkto event"=refnum} ("sweeper pair"), "talkto event"=w2, "talkback event"=w8) -> (w9:T10)
  n4 = Create User Event(user event datatype=w33) -> (user event=w26:refnum<user-event>)  [unwired: 1 in, 1 out]
  n5 = Create User Event(user event datatype=w34) -> (user event=w3:refnum<user-event>)  [unwired: 1 in, 1 out]
  n6 = Create User Event(user event datatype=w35) -> (user event=w31:refnum<user-event>)  [unwired: 1 in, 1 out]
  n7 = Create User Event(user event datatype=w36) -> (user event=w4:refnum<user-event>)  [unwired: 1 in, 1 out]
  n8 = Bundle By Name(cluster=w40, "talkto event"=w3, "talkback event"=w26) -> (w37:T10)
  n9 = Bundle By Name(cluster=w39, "talkto event"=w4, "talkback event"=w31) -> (w32:T10)
  n10 = call "gyro -- launch async sourcer.vi"("sourcer pair"=w9) -> ("reference out"=→"async sourcer":refnum<vi>, "fitter pair OUT"=w7:T10)  [unwired: 9 in]
  n11 = Create User Event(user event datatype=w28) -> (user event=w27:refnum<user-event>)  [unwired: 1 in, 1 out]
  n12 = Create User Event(user event datatype=w29) -> (user event=w5:refnum<user-event>)  [unwired: 1 in, 1 out]
  n13 = Create User Event(user event datatype=w21) -> (user event=w20:refnum<user-event>)  [unwired: 1 in, 1 out]
  n14 = Create User Event(user event datatype=w22) -> (user event=w16:refnum<user-event>)  [unwired: 1 in, 1 out]
  n15 = Bundle By Name(cluster=w30, "talkto event"=w5, "talkback event"=w27) -> (w19:T10)
  n16 = call "gyro -- launch async fitter.vi"("fitter pair"=w37) -> ("reference out"=→"async fitter":refnum<vi>, "fitter pair OUT"=w24:T10)  [unwired: 9 in]
  "fitter event pair" <- w24
  n17 = call "gyro -- launch async sweeper.vi"("sweeper event pair"=w32) -> ("reference out"=→"async sweeper":refnum<vi>, "sweeper event pair OUT"=w25:T10)  [unwired: 9 in]
  "sweeper event pair" <- w25
  n18 = Bundle By Name(cluster=w23, "talkto event"=w16, "talkback event"=w20) -> (w18:T10)
  "pll event pair" <- w18
  n19 = Unbundle By Name(w7) -> ("talkto event"=w6:refnum<user-event>)
  n20 = call "gyro -- launch async sweeper server.vi"("fitter event pair"=w24, "async sweeper event pair"=w25, "sweeper server event pair"=w19) -> ("reference out"=→"sweeper server reference":refnum<vi>)  [unwired: 8 in]
  n21 = call "gyro -- launch async pll.vi"("pll event pair"=w18) -> ("reference out"=→"pll async reference":refnum<vi>)  [unwired: 10 in]
  n22 = Generate User Event(user event=w16, event data cluster=T12 {"message"=enum."start"} ("event data")) -> (user event out=w14:refnum<user-event>)  [unwired: 2 in, 1 out]
  n23 = Create User Event(user event datatype=w43) -> (user event=w1:refnum<user-event>)  [unwired: 1 in, 1 out]
  n24 = register-events(w27, w20, w1) -> (reference out=w45:refnum<event-registration>)  [unwired: 2 in, 1 out]
  n25 = register-events(w1) -> (reference out=w51:refnum<event-registration>)  [unwired: 2 in, 1 out]
  n26 = call "aggregator - vii - real - atomic.vi"("aggregator action"=agregator_--_action."empty!", "requested size"=100, "state IN"=T14 {"requested size"=20, "Array"=[], "actual number of elements"=0}) -> ("state OUT"=w46:T14)  [unwired: 5 in, 3 out]
  n27 = while {
    shift-right: [w54] -> _
    shift-left: w46 -> [w57]
    shift-right: [w55] -> _
    shift-left: w46 -> [w56]
    tunnel: w45 -> [w53]
    tunnel: w6 -> [_]
    stop <- w52 stop-if-true
    n28 = event shown="[0] <pll talkback >: User Event" {
      selector: w53 -> [_ _]
      dyn-events: _ -> [_ _]
      timeout: _ -> [_ _]
      tunnel: w57 -> [w62 w135]
      tunnel: w56 -> [w61 w134]
      tunnel: [w60 w134] -> w55
      tunnel: [w59 w135] -> w54
      tunnel: [_ w132] -> w52
      event User Event {
        n29 = event-data() -> ("message"=w58:enum16{"new", "void"})  [unwired: 1 in]
        n30 = case shown="\"void\", Default" w58 {
          tunnel: w62 -> [w64 w124]
          tunnel: w61 -> [w63 w121]
          tunnel: [w63 w120] -> w60
          tunnel: [w64 w91] -> w59
          frame "void", Default {
          }
          frame "new" {
            w78 = 0.0 ("new X")
            n31 = call "publish -- pll result.vi"("publisher action"=publisher_action."get") -> ("pll result OUT"=w69:T19)  [unwired: 10 in]
            n32 = local read "lorentzian"() -> (w87:T5)
            n33 = Unbundle By Name(w69) -> ("freq (Hz)"=w68:dbl, "gamma (Hz)"=w67:dbl, "Voltage (V)"=w66:cdb)
            "f (Hz)" <- w68
            "G (Hz)" <- w67
            n34 = local read "plot hist time (sec)"() -> (w85:dbl)
            n35 = local read "dt (sec)"() -> (w86:dbl)
            n36 = control-ref of="Plot: complex plane"() -> (w65:refnum<vi>)
            n37 = Divide(x=w85, y=w86) -> (x/y=w115:dbl)
            n38 = Bundle By Name(cluster=T8 {"freq (Hz)"=0.0, "gamma (Hz)"=0.0, "Voltage (V)"=0.0+0.0i} ("publish message"), "freq (Hz)"=w68, "gamma (Hz)"=w67, "Voltage (V)"=w66) -> (→"publish message":T8)
            n39 = Round To Nearest(number=w115) -> (nearest integer value=w114:dbl)
            n40 = disable-structure shown="Enabled" {
              disable-tunnel: [w129 w131] -> w125
              disable-tunnel: w87 -> [w127 w130]
              disable-tunnel: [w126 w130] -> w89
              frame Disabled {
                n41 = call "lorentzian transformations.vi"("4 corner circle transformation"=four-corner_circle_transformation."get4corners", "lorentzian in"=w127) -> ("lorentzian out"=w126:T5, "4corners our"=w129:T6)  [unwired: 6 in, 2 out]
              }
              frame Enabled {
                n42 = Unbundle By Name(w130) -> ("4corners"=w131:T6)
              }
            }
            n43 = To Long Integer(number=w114) -> (32bit integer=w113:i32)
            n44 = call "aggregator - vii - complex - atomic.vi"("aggregator action"=agregator_--_action."append", "requested size"=w113, "state IN"=w124) -> ("state OUT"=w91:T20)  [unwired: 5 in, 3 out]
            n45 = Complex To Re/Im(x + iy=w66) -> (x=→"zi out Re (V)":dbl, y=→"zi out Im (V)":dbl)
            n46 = call "aggregator - vii - real - atomic.vi"("aggregator action"=agregator_--_action."append", "requested size"=w113, "state IN"=w121) -> ("state OUT"=w120:T14)  [unwired: 5 in, 3 out]
            n47 = Complex To Re/Im(x + iy=w66) -> (x=w82:dbl, y=w83:dbl)
            n48 = call "draw complex lorentzian.vi"("4 corners"=w125) -> ("fancy circles"=→"Plot: complex plane":cluster{dbl[], dbl[]}[])  [unwired: 10 in]
            n49 = call "replace cursor - plot ref - V2.vi"("Plot ref in"=w65, "new X"=w82, "new  Y"=w83, "cursor index"=0, "cursor action"=cursor_action."write", "Color Box"=u32 327424) -> ("Plot ref out"=w84:refnum<vi>)  [unwired: 10 in, 3 out]
            n50 = Unbundle By Name(w120) -> ("Array"=w107:dbl[])
            n51 = Unbundle By Name(w91) -> ("Array"=w108:cdb[])
            n52 = call "replace cursor - plot ref - V2.vi"("Plot ref in"=w84, "new X"=w78, "new  Y"=w78, "cursor index"=1, "cursor action"=cursor_action."write", "Color Box"=u32 5880319) -> ()  [unwired: 10 in, 4 out]
            n53 = call "linear interp iiii- complex - z-omega.vi"("z"=w108, "omega"=w107) -> ("slope"=w106:cdb)  [unwired: 5 in, 8 out]
            n54 = Unbundle By Name(w89) -> ("4corners.z center"=w88:cdb, "A (VHz)"=w101:dbl, "G (Hz)"=w103:dbl)
            n55 = Complex To Polar(r * e^(i*theta)=w106) -> (r=w105:dbl)  [unwired: 1 out]
            n56 = Divide(x=w106, y=w105) -> (x/y=w104:cdb)
            n57 = call "lorentzian transformations.vi"("4 corner circle transformation"=four-corner_circle_transformation."get4corners", "lorentzian in"="lorentzian -- hist") -> ("4corners our"=w112:T6)  [unwired: 6 in, 3 out]
            n58 = Reciprocal(x=w103) -> (1/x=w102:dbl)
            n59 = Complex To Re/Im(x + iy=w108) -> (x=w118:dbl[], y=w117:dbl[])
            n60 = Compound Arithmetic op=MULTIPLY(w104, w102, w101, 1.1 ("value")) -> (w94:cdb)
            n61 = call "draw complex lorentzian.vi"("4 corners"=w112) -> ("fancy circles"=w110:cluster{dbl[], dbl[]}[])  [unwired: 10 in]
            n62 = Bundle(w118, w117) -> (w119:cluster{dbl[], dbl[]})  [unwired: 1 in]
            n63 = Add(x=w88, y=w94) -> (x+y=w100:cdb)
            n64 = Subtract(x=w88, y=w94) -> (x-y=w99:cdb)
            n65 = Complex To Re/Im(x + iy=w100) -> (x=w98:dbl, y=w96:dbl)
            n66 = Complex To Re/Im(x + iy=w99) -> (x=w97:dbl, y=w95:dbl)
            n67 = call "draw a line.vi"("y1"=w95, "y0"=w96, "x1"=w97, "x0"=w98) -> ("output cluster"=w92:cluster{dbl[], dbl[]})  [unwired: 7 in]
            n68 = Build Array (concatenate)(w119, w110, w92) -> (→"Plot: complex- hist":cluster{dbl[], dbl[]}[])
          }
        }
      }
      event User Event {
        n69 = event-data() -> ("pll internal user event action"=w133:T13)  [unwired: 1 in]
        n70 = case shown="\"void\", Default" w133 {
          tunnel: [_ TRUE] -> w132
          frame "void", Default {
          }
          frame "exit" {
          }
        }
      }
    }
  }
  n71 = control-ref of="Plot: complex- hist"() -> (w47:refnum<vi>)
  n72 = control-ref of="Plot: complex plane"() -> (w44:refnum<vi>)
  n73 = while {
    tunnel: w51 -> [w146]
    tunnel: w1 -> [w145]
    tunnel: w44 -> [w144]
    tunnel: w47 -> [w143]
    tunnel: w14 -> [w142]
    tunnel: w19 -> [_]
    tunnel: w5 -> [w141]
    tunnel: w4 -> [w140]
    tunnel: w3 -> [w139]
    tunnel: w2 -> [w138]
    stop <- w137 stop-if-true
    n74 = event shown="[0] <pll internal user event action>: User Event" {
      selector: w146 -> [_ _ _ _ _ _ _ _ _ _ _ _ _ _ _ _]
      dyn-events: _ -> [_ _ _ _ _ _ _ _ _ _ _ _ _ _ _ _]
      timeout: _ -> [_ _ _ _ _ _ _ _ _ _ _ _ _ _ _ _]
      tunnel: [_ "(*) pll" "(*) sourcer" "(*) fitter" "(*) sweeper" "(*) sweeper server" "exit!" "stop pll async" "start pll async" "toggle PLL! :@" _ "reset freq! :r" "reset lorentzian! :q" "reset lorentzian from basic" "save lor for later" _] -> _
      tunnel: w145 -> [w153 w238 w241 w244 w247 w250 w252 w256 w259 w262 _ w297 w300 _ _ w311]
      tunnel: w144 -> [w154 _ _ _ _ _ _ _ _ _ w268 _ _ _ _ w310]
      tunnel: w143 -> [_ _ _ _ _ _ _ _ _ _ _ _ _ _ _ w309]
      tunnel: w142 -> [w152 _ _ _ _ _ _ _ _ _ _ _ _ _ _ _]
      tunnel: w141 -> [w151 _ _ _ _ _ _ _ _ _ _ _ _ _ _ _]
      tunnel: w140 -> [w150 _ _ _ _ _ _ _ _ _ _ _ _ _ _ _]
      tunnel: w139 -> [w149 _ _ _ _ _ _ _ _ _ _ _ _ _ _ _]
      tunnel: w138 -> [w148 _ _ _ _ _ _ _ _ _ _ _ _ _ _ _]
      tunnel: [w147 _ _ _ _ _ _ _ _ _ _ _ _ _ _ _] -> w137
      event User Event {
        n75 = event-data() -> ("pll internal user event action"=w155:T13)  [unwired: 1 in]
        n76 = case shown="\"gear pll async\"" w155 {
          tunnel: w154 -> [_ _ _ _ _ _ _ _ _ _ _ _ w230 _]
          tunnel: w153 -> [_ _ w160 _ _ w173 _ _ _ _ _ w214 _ w232]
          tunnel: w152 -> [_ w157 w165 w168 w169 w180 _ _ _ _ _ _ _ _]
          tunnel: w151 -> [_ _ _ _ _ w179 _ _ _ _ _ _ _ _]
          tunnel: w150 -> [_ _ _ _ _ w178 _ _ _ _ _ _ _ _]
          tunnel: w149 -> [_ _ _ _ _ w177 _ _ _ _ _ _ _ _]
          tunnel: w148 -> [_ _ _ _ _ w176 _ _ _ _ _ _ _ _]
          tunnel: [_ _ _ _ _ TRUE _ _ _ _ _ _ _ _] -> w147
          frame "void", Default {
          }
          frame "accept frequency" {
            n77 = Generate User Event(user event=w157, event data cluster=T12 {"message"=enum."reset"} ("event data")) -> ()  [unwired: 2 in, 2 out]
          }
          frame "accept lorentzian" {
            n78 = Generate User Event(user event=w160, event data cluster=pll_internal_user_event_action."update cursors" ("event data")) -> ()  [unwired: 2 in, 2 out]
            n79 = call "publish -- lorentzian.vi"("publisher action"=publisher_action."get") -> ("lorentzian OUT"=w164:T5)  [unwired: 10 in]
            n80 = Generate User Event(user event=w165, event data cluster=T12 {"message"=enum."update request"} ("event data")) -> ()  [unwired: 2 in, 2 out]
            n81 = call "lorentzian transformations.vi"("4 corner circle transformation"=four-corner_circle_transformation."get4corners", "lorentzian in"=w164) -> ("lorentzian out"=w163:T5)  [unwired: 6 in, 3 out]
            n82 = local write "lorentzian -- hist"(w163) -> ()
            n83 = local write "lorentzian"(w163) -> ()
          }
          frame "pause pll" {
            n84 = Generate User Event(user event=w168, event data cluster=T12 {"message"=enum."pause"} ("event data")) -> ()  [unwired: 2 in, 2 out]
            n85 = local write "PLL ON"(FALSE ("PLL ON")) -> ()
          }
          frame "start pll async" {
            n86 = Generate User Event(user event=w169, event data cluster=T12 {"message"=enum."unpause"} ("event data")) -> ()  [unwired: 2 in, 2 out]
            n87 = local write "PLL ON"(TRUE ("PLL ON")) -> ()
          }
          frame "exit" {
            w175 = T12 {"message"=enum."exit"} ("event data")
            n88 = Generate User Event(user event=w173, event data cluster=pll_internal_user_event_action."exit" ("event data")) -> ()  [unwired: 2 in, 2 out]
            n89 = Generate User Event(user event=w180, event data cluster=w175) -> ()  [unwired: 2 in, 2 out]
            n90 = Generate User Event(user event=w177, event data cluster=w175) -> ()  [unwired: 2 in, 2 out]
            n91 = Generate User Event(user event=w176, event data cluster=w175) -> ()  [unwired: 2 in, 2 out]
            n92 = Generate User Event(user event=w178, event data cluster=w175) -> ()  [unwired: 2 in, 2 out]
            n93 = Generate User Event(user event=w179, event data cluster=w175) -> ()  [unwired: 2 in, 2 out]
            n94 = local write "PLL ON"(FALSE ("PLL ON")) -> ()
          }
          frame "gear pll async" {
            n95 = local read "pll async reference"() -> (w183:refnum<vi>)
            n96 = property class="VI Interface Type 3"(reference=w183) -> ("FP.State"=w182:T21)  [unwired: 1 in, 2 out]
            n97 = case shown="\"Standard\", Default" w182 {
              tunnel: w183 -> [w186 w187]
              frame "Closed" {
                n98 = invoke class="VI (strict)" method="FP.Open"(reference=w186, "Activate"=TRUE ("Activate?"), "State"=T21."Standard" ("Front Panel Window:State")) -> ()  [unwired: 2 in, 5 out]
              }
              frame "Standard", Default {
                n99 = invoke class="VI (strict)" method="FP.Close"(reference=w187) -> ()  [unwired: 2 in, 3 out]
              }
            }
          }
          frame "gear server sweeper" {
            n100 = local read "sweeper server reference"() -> (w189:refnum<vi>)
            n101 = property class="VI Interface Type 2"(reference=w189) -> ("FP.State"=w188:T21)  [unwired: 1 in, 2 out]
            n102 = case shown="\"Standard\", Default" w188 {
              tunnel: w189 -> [w192 w193]
              frame "Closed" {
                n103 = invoke class="VI (strict)" method="FP.Open"(reference=w192, "Activate"=TRUE ("Activate?"), "State"=T21."Standard" ("Front Panel Window:State")) -> ()  [unwired: 2 in, 5 out]
              }
              frame "Standard", Default {
                n104 = invoke class="VI (strict)" method="FP.Close"(reference=w193) -> ()  [unwired: 2 in, 3 out]
              }
            }
          }
          frame "gear sweeper async" {
            n105 = local read "async sweeper"() -> (w195:refnum<vi>)
            n106 = property class="VI Interface Type 3"(reference=w195) -> ("FP.State"=w194:T21)  [unwired: 1 in, 2 out]
            n107 = case shown="\"Standard\", Default" w194 {
              tunnel: w195 -> [w198 w199]
              frame "Closed" {
                n108 = invoke class="VI (strict)" method="FP.Open"(reference=w198, "Activate"=TRUE ("Activate?"), "State"=T21."Standard" ("Front Panel Window:State")) -> ()  [unwired: 2 in, 5 out]
              }
              frame "Standard", Default {
                n109 = invoke class="VI (strict)" method="FP.Close"(reference=w199) -> ()  [unwired: 2 in, 3 out]
              }
            }
          }
          frame "gear fitter" {
            n110 = local read "async fitter"() -> (w201:refnum<vi>)
            n111 = property class="VI Interface Type 3"(reference=w201) -> ("FP.State"=w200:T21)  [unwired: 1 in, 2 out]
            n112 = case shown="\"Standard\", Default" w200 {
              tunnel: w201 -> [w204 w205]
              frame "Closed" {
                n113 = invoke class="VI (strict)" method="FP.Open"(reference=w204, "Activate"=TRUE ("Activate?"), "State"=T21."Standard" ("Front Panel Window:State")) -> ()  [unwired: 2 in, 5 out]
              }
              frame "Standard", Default {
                n114 = invoke class="VI (strict)" method="FP.Close"(reference=w205) -> ()  [unwired: 2 in, 3 out]
              }
            }
          }
          frame "gear sourcer" {
            n115 = local read "async sourcer"() -> (w207:refnum<vi>)
            n116 = property class="VI Interface Type 3"(reference=w207) -> ("FP.State"=w206:T21)  [unwired: 1 in, 2 out]
            n117 = case shown="\"Standard\", Default" w206 {
              tunnel: w207 -> [w210 w211]
              frame "Closed" {
                n118 = invoke class="VI (strict)" method="FP.Open"(reference=w210, "Activate"=TRUE ("Activate?"), "State"=T21."Standard" ("Front Panel Window:State")) -> ()  [unwired: 2 in, 5 out]
              }
              frame "Standard", Default {
                n119 = invoke class="VI (strict)" method="FP.Close"(reference=w211) -> ()  [unwired: 2 in, 3 out]
              }
            }
          }
          frame "toggle pll async" {
            n120 = local read "PLL ON"() -> (w213:bool)
            n121 = case shown="True" w213 {
              tunnel: [pll_internal_user_event_action."unpause pll" ("event data") pll_internal_user_event_action."pause pll" ("event data")] -> w212
              frame False {
              }
              frame True {
              }
            }
            n122 = Generate User Event(user event=w214, event data cluster=w212) -> ()  [unwired: 2 in, 2 out]
          }
          frame "update cursors" {
            n123 = local read "lorentzian"() -> (w217:T5)
            n124 = Unbundle By Name(w217) -> ("4corners.z(inf)"=w225:cdb, "4corners.z(0)"=w218:cdb)
            n125 = Complex To Re/Im(x + iy=w225) -> (x=w227:dbl, y=w226:dbl)
            n126 = Complex To Re/Im(x + iy=w218) -> (x=w221:dbl, y=w220:dbl)
            n127 = call "replace cursor - plot ref - V2.vi"("Plot ref in"=w230, "new X"=w227, "new  Y"=w226, "cursor index"=2, "cursor action"=cursor_action."write", "Color Box"=u32 16746738) -> ()  [unwired: 10 in, 4 out]
            n128 = call "replace cursor - plot ref - V2.vi"("Plot ref in"=w230, "new X"=w221, "new  Y"=w220, "cursor index"=3, "cursor action"=cursor_action."write", "Color Box"=u32 10682154) -> ()  [unwired: 10 in, 4 out]
          }
          frame "toggle sweeper" {
            n129 = case shown="True" "PLL ON" {
              tunnel: w232 -> [_ w234]
              frame False {
              }
              frame True {
                n130 = Generate User Event(user event=w234, event data cluster=pll_internal_user_event_action."pause pll" ("event data")) -> ()  [unwired: 2 in, 2 out]
              }
            }
            n131 = Generate User Event(user event=w232, event data cluster=pll_internal_user_event_action."start sweeper" ("event data")) -> ()  [unwired: 2 in, 2 out]
          }
        }
      }
      event "(*) pll": Value Change {
        n132 = event-data() -> ()  [unwired: 1 in, 6 out]
        n133 = Generate User Event(user event=w238, event data cluster=pll_internal_user_event_action."gear pll async" ("event data")) -> ()  [unwired: 2 in, 2 out]
      }
      event "(*) sourcer": Value Change {
        n134 = event-data() -> ()  [unwired: 1 in, 6 out]
        n135 = Generate User Event(user event=w241, event data cluster=pll_internal_user_event_action."gear sourcer" ("event data")) -> ()  [unwired: 2 in, 2 out]
      }
      event "(*) fitter": Value Change {
        n136 = event-data() -> ()  [unwired: 1 in, 6 out]
        n137 = Generate User Event(user event=w244, event data cluster=pll_internal_user_event_action."gear fitter" ("event data")) -> ()  [unwired: 2 in, 2 out]
      }
      event "(*) sweeper": Value Change {
        n138 = event-data() -> ()  [unwired: 1 in, 6 out]
        n139 = Generate User Event(user event=w247, event data cluster=pll_internal_user_event_action."gear sweeper async" ("event data")) -> ()  [unwired: 2 in, 2 out]
      }
      event "(*) sweeper server": Value Change {
        n140 = event-data() -> ()  [unwired: 1 in, 6 out]
        n141 = Generate User Event(user event=w250, event data cluster=pll_internal_user_event_action."gear server sweeper" ("event data")) -> ()  [unwired: 2 in, 2 out]
      }
      event "exit!": Value Change {
        n142 = event-data() -> ()  [unwired: 1 in, 6 out]
        n143 = Generate User Event(user event=w252, event data cluster=pll_internal_user_event_action."exit" ("event data")) -> ()  [unwired: 2 in, 2 out]
      }
      event "stop pll async": Value Change {
        n144 = event-data() -> ()  [unwired: 1 in, 6 out]
        n145 = Generate User Event(user event=w256, event data cluster=pll_internal_user_event_action."stop pll async" ("event data")) -> ()  [unwired: 2 in, 2 out]
      }
      event "start pll async": Value Change {
        n146 = event-data() -> ()  [unwired: 1 in, 6 out]
        n147 = Generate User Event(user event=w259, event data cluster=pll_internal_user_event_action."stop pll async" ("event data")) -> ()  [unwired: 2 in, 2 out]
      }
      event "toggle PLL! :@": Value Change {
        n148 = event-data() -> ()  [unwired: 1 in, 1 out]
        n149 = Generate User Event(user event=w262, event data cluster=pll_internal_user_event_action."toggle pll async" ("event data")) -> ()  [unwired: 2 in, 2 out]
      }
      event "Plot: complex plane": Cursor Move {
        n150 = event-data() -> ("CursIdx"=w267:i32)  [unwired: 1 in]
        n151 = local read "lorentzian"() -> (w266:T5)
        n152 = case shown="2" w267 {
          selector: w267 -> [_ w280 w290]
          tunnel: w268 -> [_ w274 w289]
          tunnel: w266 -> [w269 w270 w288]
          tunnel: [w269 w271 w285] -> w264
          frame 0, Default {
          }
          frame 2 {
            n153 = call "replace cursor - plot ref - V2.vi"("Plot ref in"=w274, "cursor index"=w280, "cursor action"=cursor_action."read") -> ("read X"=w282:dbl, "read Y"=w283:dbl)  [unwired: 13 in, 2 out]
            n154 = Re/Im To Complex(1:w283, 2:w282) -> (0:w281:cdb)
            n155 = Bundle By Name(cluster=w270, "bg (V)"=w281) -> (w279:T5)
            n156 = call "lorentzian transformations.vi"("4 corner circle transformation"=four-corner_circle_transformation."get4corners", "lorentzian in"=w279) -> ("lorentzian out"=w271:T5)  [unwired: 6 in, 3 out]
            n157 = Unbundle By Name(w271) -> ("4corners.z(0)"=w277:cdb)
            n158 = Complex To Re/Im(x + iy=w277) -> (x=w276:dbl, y=w275:dbl)
            n159 = call "replace cursor - plot ref - V2.vi"("Plot ref in"=w274, "new X"=w276, "new  Y"=w275, "cursor index"=3, "cursor action"=cursor_action."write") -> ()  [unwired: 11 in, 4 out]
          }
          frame 3 {
            n160 = call "replace cursor - plot ref - V2.vi"("Plot ref in"=w289, "cursor index"=w290, "cursor action"=cursor_action."read") -> ("read X"=w292:dbl, "read Y"=w293:dbl)  [unwired: 13 in, 2 out]
            n161 = Re/Im To Complex(1:w293, 2:w292) -> (0:w291:cdb)
            n162 = Bundle By Name(cluster=w288, "4corners.z(0)"=w291) -> (w287:T5)
            n163 = call "lorentzian transformations.vi"("4 corner circle transformation"=four-corner_circle_transformation."update lorentzian -- from z0", "lorentzian in"=w287) -> ("lorentzian out"=w285:T5)  [unwired: 6 in, 3 out]
          }
        }
        n164 = call "lorentzian transformations.vi"("4 corner circle transformation"=four-corner_circle_transformation."get4corners", "lorentzian in"=w264) -> ("lorentzian out"=w263:T5)  [unwired: 6 in, 3 out]
        n165 = local write "lorentzian"(w263) -> ()
      }
      event "reset freq! :r": Value Change {
        n166 = event-data() -> ()  [unwired: 1 in, 6 out]
        n167 = Generate User Event(user event=w297, event data cluster=pll_internal_user_event_action."accept frequency" ("event data")) -> ()  [unwired: 2 in, 2 out]
      }
      event "reset lorentzian! :q": Value Change {
        n168 = event-data() -> ()  [unwired: 1 in, 6 out]
        n169 = Generate User Event(user event=w300, event data cluster=pll_internal_user_event_action."accept lorentzian" ("event data")) -> ()  [unwired: 2 in, 2 out]
      }
      event "reset lorentzian from basic": Value Change {
        n170 = event-data() -> ()  [unwired: 1 in, 6 out]
        n171 = local read "lorentzian -- basic"() -> (w302:T5)
        n172 = call "lorentzian transformations.vi"("4 corner circle transformation"=four-corner_circle_transformation."get4corners", "lorentzian in"=w302) -> ("lorentzian out"=w301:T5)  [unwired: 6 in, 3 out]
        n173 = local write "lorentzian"(w301) -> ()
      }
      event "save lor for later": Value Change {
        n174 = event-data() -> ()  [unwired: 1 in, 6 out]
        n175 = local read "lorentzian"() -> (w306:T5)
        n176 = call "lorentzian transformations.vi"("4 corner circle transformation"=four-corner_circle_transformation."get4corners", "lorentzian in"=w306) -> ("lorentzian out"=w305:T5)  [unwired: 6 in, 3 out]
        n177 = local write "lorentzian -- basic"(w305) -> ()
      }
      event Key Down {
        n178 = event-data() -> ("Char"=w313:i16, "VKey"=w315:T7)  [unwired: 1 in]
        "Char" <- w313
        "VKey" <- w315
        n179 = Build Array(w313) -> (w314:i16[])
        n180 = Byte Array To String(unsigned byte array=w314) -> (string=w312:string)
        n181 = case shown="\"ASCII\", Default" w315 {
          selector: w315 -> [_ _ _ _ w398]
          tunnel: w313 -> [_ _ _ _ _]
          tunnel: w312 -> [w319 _ _ _ _]
          tunnel: w311 -> [w318 _ _ _ _]
          tunnel: w310 -> [w317 _ _ _ w397]
          tunnel: w309 -> [w316 _ _ _ w396]
          frame "ASCII", Default {
            n182 = case shown="\"q\"" w319 {
              selector: w319 -> [_ w322 _ w332 _ _ _]
              tunnel: w318 -> [_ _ w330 _ w390 w392 w394]
              tunnel: w317 -> [_ w321 _ _ _ _ _]
              tunnel: w316 -> [_ w320 _ _ _ _ _]
              frame "0", Default {
              }
              frame "<", ">", "?", "A", "z" {
                n183 = case shown="\"A\"" w322 {
                  tunnel: [cursor_action."zoom out 20%" ("cursor action") cursor_action."zoom in 20%" ("cursor action") cursor_action."smart zoom out&aspect" ("cursor action") cursor_action."smart zoom out" ("cursor action") cursor_action."zoom to aspect ratio 1" ("cursor action")] -> w323
                  frame ">" {
                  }
                  frame "<" {
                  }
                  frame "?" {
                  }
                  frame "A" {
                  }
                  frame "z", Default {
                  }
                }
                n184 = call "replace cursor - plot ref - V2.vi"("Plot ref in"=w321, "cursor action"=w323) -> ()  [unwired: 14 in, 4 out]
                n185 = call "replace cursor - plot ref - V2.vi"("Plot ref in"=w320, "cursor action"=w323) -> ()  [unwired: 14 in, 4 out]
              }
              frame "r" {
                (unwired) "reset frequency" ("event data")
                n186 = Generate User Event(user event=w330, event data cluster=pll_internal_user_event_action."accept frequency" ("event data")) -> ()  [unwired: 2 in, 2 out]
              }
              frame "'", ";", "[", "]", "{", "}" {
                n187 = control-ref of="PID parameters :{}[];'"() -> (w331:refnum<vi>)
                n188 = case shown="\"]\"" w332 {
                  tunnel: w331 -> [w337 w346 w355 w364 w373 w383]
                  frame "[" {
                    n189 = property class="Clust (strict)"(reference=w337) -> (reference out=w336:refnum<vi>, "Value"=w335:T1)  [unwired: 1 in, 1 out]
                    n190 = in-place {
                      in-place-border: 0.9 -> [w340]
                      n191 = in-place-cluster #1(w335) -> ("P (sec)"=w338:dbl, "I (sec)"=w341:dbl)
                      n192 = Multiply(x=w341, y=w340) -> (x*y=w339:dbl)
                      n193 = in-place-cluster #1("P (sec)"=w338, "I (sec)"=w339) -> (w334:T1)
                    }
                    n194 = property class="Clust (strict)"(reference=w336, "Value"=w334) -> ()  [unwired: 1 in, 2 out]
                  }
                  frame "]" {
                    n195 = property class="Clust (strict)"(reference=w346) -> (reference out=w345:refnum<vi>, "Value"=w344:T1)  [unwired: 1 in, 1 out]
                    n196 = in-place {
                      in-place-border: 1.1 -> [w349]
                      n197 = in-place-cluster #2(w344) -> ("P (sec)"=w347:dbl, "I (sec)"=w350:dbl)
                      n198 = Multiply(x=w350, y=w349) -> (x*y=w348:dbl)
                      n199 = in-place-cluster #2("P (sec)"=w347, "I (sec)"=w348) -> (w343:T1)
                    }
                    n200 = property class="Clust (strict)"(reference=w345, "Value"=w343) -> ()  [unwired: 1 in, 2 out]
                  }
                  frame "}" {
                    n201 = property class="Clust (strict)"(reference=w355) -> (reference out=w354:refnum<vi>, "Value"=w353:T1)  [unwired: 1 in, 1 out]
                    n202 = in-place {
                      in-place-border: 1.1 -> [w359]
                      n203 = in-place-cluster #3(w353) -> ("P (sec)"=w358:dbl, "I (sec)"=w356:dbl)
                      n204 = Multiply(x=w358, y=w359) -> (x*y=w357:dbl)
                      n205 = in-place-cluster #3("P (sec)"=w357, "I (sec)"=w356) -> (w352:T1)
                    }
                    n206 = property class="Clust (strict)"(reference=w354, "Value"=w352) -> ()  [unwired: 1 in, 2 out]
                  }
                  frame "{", Default {
                    n207 = property class="Clust (strict)"(reference=w364) -> (reference out=w363:refnum<vi>, "Value"=w362:T1)  [unwired: 1 in, 1 out]
                    n208 = in-place {
                      in-place-border: 0.9 -> [w368]
                      n209 = in-place-cluster #4(w362) -> ("P (sec)"=w367:dbl, "I (sec)"=w365:dbl)
                      n210 = Multiply(x=w367, y=w368) -> (x*y=w366:dbl)
                      n211 = in-place-cluster #4("P (sec)"=w366, "I (sec)"=w365) -> (w361:T1)
                    }
                    n212 = property class="Clust (strict)"(reference=w363, "Value"=w361) -> ()  [unwired: 1 in, 2 out]
                  }
                  frame "'" {
                    n213 = property class="Clust (strict)"(reference=w373) -> (reference out=w372:refnum<vi>, "Value"=w371:T1)  [unwired: 1 in, 1 out]
                    n214 = in-place {
                      in-place-border: 1.1 -> [w374]
                      n215 = in-place-cluster #5(w371) -> ("P (sec)"=w378:dbl, "I (sec)"=w376:dbl)
                      n216 = Multiply(x=w378, y=w374) -> (x*y=w377:dbl)
                      n217 = Multiply(x=w376, y=w374) -> (x*y=w375:dbl)
                      n218 = in-place-cluster #5("P (sec)"=w377, "I (sec)"=w375) -> (w370:T1)
                    }
                    n219 = property class="Clust (strict)"(reference=w372, "Value"=w370) -> ()  [unwired: 1 in, 2 out]
                  }
                  frame ";" {
                    n220 = property class="Clust (strict)"(reference=w383) -> (reference out=w382:refnum<vi>, "Value"=w381:T1)  [unwired: 1 in, 1 out]
                    n221 = in-place {
                      in-place-border: 0.9 -> [w384]
                      n222 = in-place-cluster #6(w381) -> ("P (sec)"=w388:dbl, "I (sec)"=w386:dbl)
                      n223 = Multiply(x=w388, y=w384) -> (x*y=w387:dbl)
                      n224 = Multiply(x=w386, y=w384) -> (x*y=w385:dbl)
                      n225 = in-place-cluster #6("P (sec)"=w387, "I (sec)"=w385) -> (w380:T1)
                    }
                    n226 = property class="Clust (strict)"(reference=w382, "Value"=w380) -> ()  [unwired: 1 in, 2 out]
                  }
                }
              }
              frame "@" {
                (unwired) "toggle PLL" ("event data")
                n227 = Generate User Event(user event=w390, event data cluster=pll_internal_user_event_action."toggle pll async" ("event data")) -> ()  [unwired: 2 in, 2 out]
              }
              frame "#" {
                (unwired) "(sweeper) sweep!" ("event data")
                n228 = Generate User Event(user event=w392, event data cluster=pll_internal_user_event_action."toggle sweeper" ("event data")) -> ()  [unwired: 2 in, 2 out]
              }
              frame "q" {
                (unwired) "reset lorentzian" ("event data")
                n229 = Generate User Event(user event=w394, event data cluster=pll_internal_user_event_action."accept lorentzian" ("event data")) -> ()  [unwired: 2 in, 2 out]
              }
            }
          }
          frame "Escape" {
          }
          frame "PageUp" {
          }
          frame "PageDown" {
          }
          frame "Up".."Right" {
            n230 = case shown="\"Down\"" w398 {
              tunnel: [cursor_action."move range right 20%" ("cursor action") cursor_action."move range left 20%" ("cursor action") cursor_action."move range up 20%" ("cursor action") cursor_action."move range down 20%" ("cursor action")] -> w395
              frame "Right", Default {
              }
              frame "Left" {
              }
              frame "Up" {
              }
              frame "Down" {
              }
            }
            n231 = call "replace cursor - plot ref - V2.vi"("Plot ref in"=w397, "cursor action"=w395) -> ()  [unwired: 14 in, 4 out]
            n232 = call "replace cursor - plot ref - V2.vi"("Plot ref in"=w396, "cursor action"=w395) -> ()  [unwired: 14 in, 4 out]
          }
        }
      }
    }
  }
  n233 = while {
    stop <- FALSE stop-if-true
    n234 = local read "publish message"() -> (w407:T8)
    n235 = Unbundle By Name(w407) -> ("freq (Hz)"=w406:dbl, "Voltage (V)"=w405:cdb, "gamma (Hz)"=w404:dbl)
    n236 = Wait (ms)(milliseconds to wait=u32 30) -> ()  [unwired: 1 out]
    n237 = call "publish -- get frequency and voltage.vi"("publisher action"=publisher_action."set", "gamma IN (Hz)"=w404, "Voltage IN (V)"=w405, "freq IN (Hz)"=w406) -> ()  [unwired: 5 in, 3 out]
  }
